vi "New Targets Info.vi"(1 "Z":dbl, 2 "Y":dbl) -> (0 "Target Info":cluster{"X":dbl, "Y":dbl, "Z":dbl})   [LabVIEW 2016]
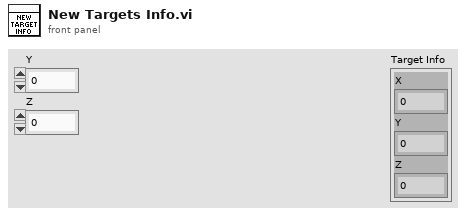
[diagram p1: front panel]
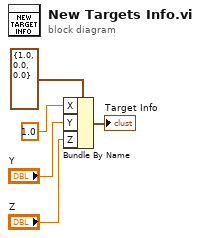
[diagram p0: block diagram]
diagram:
  n1 = Bundle By Name(cluster=cluster{"X":dbl, "Y":dbl, "Z":dbl} {"X"=1.0, "Y"=0.0, "Z"=0.0}, "X"=1.0, "Y"="Y", "Z"="Z") -> (→"Target Info":cluster{"X":dbl, "Y":dbl, "Z":dbl})
